vi "Refresh and Highlight Item.vi"(5 "Project Name":string, 7 "Section":string, 8 "error in":errorcluster, 9 "Item name":string, 10 "Library Name":string, 11 "Delacor_lib_QMH_Message Queue in":refnum<class "Delacor_lib_QMH_Message Queue.lvclass">) -> (0 "error out":errorcluster)   [LabVIEW 2019, in "Panther Dashboard.lvlib"]
uses:
  Panther Dashboard.lvlib
  <vilib>/Delacor/Delacor QMH/Libraries/Message Queue_class/Delacor_lib_QMH_Message Queue.lvclass
  <vilib>/Delacor/Delacor QMH/Libraries/Message Queue_class/Delacor_lib_QMH_Message Queue.lvclass/Delacor_lib_QMH_Message Queue.ctl
  <vilib>/Delacor/Delacor QMH/Libraries/Message Queue_class/Delacor_lib_QMH_Enqueue Message (Single).vi
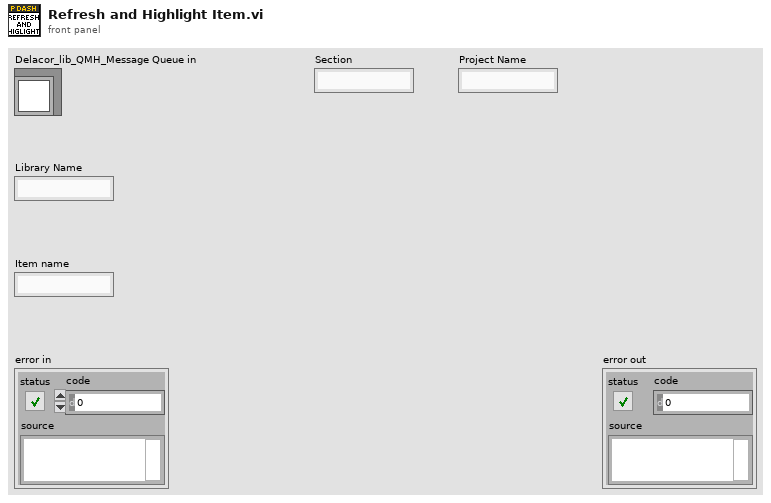
[diagram p1: front panel]
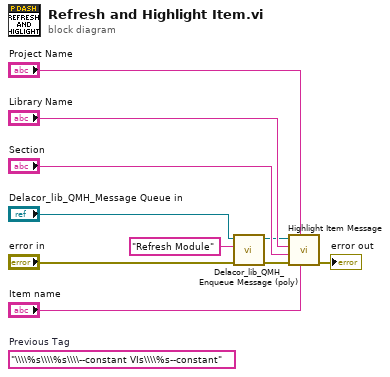
[diagram p0: block diagram]
diagram:
  (unwired) "\\\\%s\\\\%s\\\\--constant VIs\\\\%s--constant"  # Previous Tag
  n1 = call-poly <vilib>:"Delacor_lib_QMH_Enqueue Message (poly).vi"("error in"="error in", "Message"="Refresh Module", "Message Queue in"="Delacor_lib_QMH_Message Queue in") -> ("error out"=w8:errorcluster, "Message Queue out"=w1:refnum<class "Delacor_lib_QMH_Message Queue.lvclass">)  [unwired: 7 in]
  n2 = call "Highlight Item Message.vi"("Item name"="Item name", "Project Name"="Project Name", "error in (no error)"=w8, "Section"="Section", "Library Name"="Library Name", "Delacor_lib_QMH_Message Queue in"=w1) -> ("error out"=→"error out":errorcluster)  [unwired: 5 in]
